vi "Read File.vi"(8 "error in (no error)":errorcluster, 11 "DAT in":refnum<class "Data.DAT.lvclass">) -> (0 "error out":errorcluster, 3 "DAT out":refnum<class "Data.DAT.lvclass">)   [LabVIEW 2016, in "Data.DAT.lvclass"]
uses:
  Data.DAT.lvclass
  C:/user/patrick/git/LV-to-ITX/src/Data/Data.lvclass
  Data/Data.lvclass/Data.ctl
  <vilib>/Utility/file.llb/Read Delimited Spreadsheet (string).vi
  Data/Data.lvclass
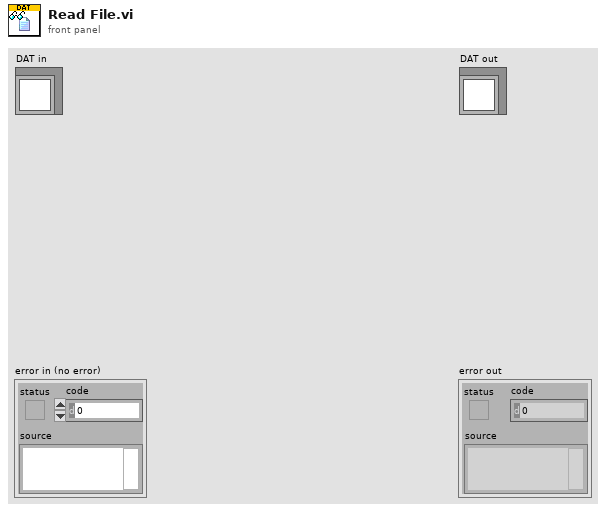
[diagram p1: front panel]
types:
  T1 = typedef "Data.lvclass/Dictionary--cluster.ctl" = cluster{"key":string, "value":variant}
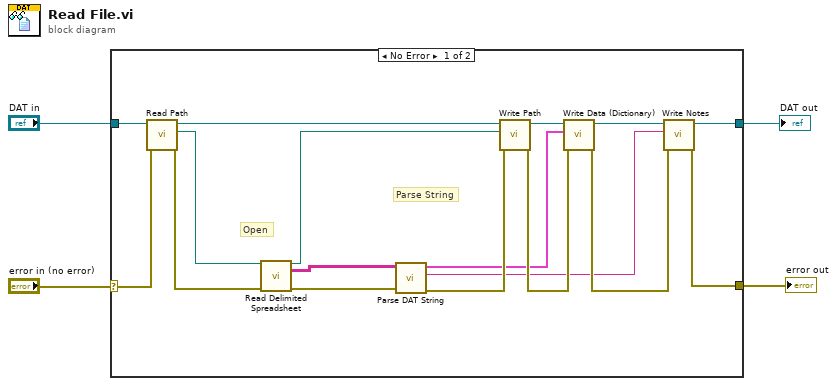
[diagram p0: block diagram]
diagram:
  n1 = case shown="No Error" "error in (no error)" {
    selector: "error in (no error)" -> [w5 w23]
    tunnel: "DAT in" -> [w8 w22]
    tunnel: [w7 w22] -> w3
    tunnel: [w6 w23] -> w2
    frame No Error {
      # "Parse String"
      # "Open"
      n2 = call "Read Path.vi"("error in (no error)"=w5, "Data Save"=w8) -> ("error out"=w20:errorcluster, "Path"=w10:path, "Data Save out"=w19:refnum<class "Data.DAT.lvclass">)  [unwired: 7 in]
      n3 = call-poly <vilib>:"Read Delimited Spreadsheet.vi"("file path (dialog if empty)"=w10, "error in (no error)"=w20) -> ("new file path (Not A Path if cancelled)"=w11:path, "all rows"=w9:string[][], "error out"=w21:errorcluster)  [unwired: 8 in, 3 out]
      n4 = call "Parse DAT String.vi"("error in (no error)"=w21, "spreadsheet string"=w9) -> ("error out"=w14:errorcluster, "Notes"=w12:string, "Data (Dictionary)"=w13:T1[])  [unwired: 7 in]
      n5 = call "Write Path.vi"("error in (no error)"=w14, "Path"=w11, "Data Save"=w19) -> ("error out"=w16:errorcluster, "Data Save out"=w18:refnum<class "Data.DAT.lvclass">)  [unwired: 7 in]
      n6 = call "Write Data (Dictionary).vi"("error in (no error)"=w16, "Data (Dictionary)"=w13, "Data Save"=w18) -> ("error out"=w15:errorcluster, "Data Save out"=w17:refnum<class "Data.DAT.lvclass">)  [unwired: 7 in]
      n7 = call "Write Notes.vi"("error in (no error)"=w15, "Notes"=w12, "Data Save"=w17) -> ("error out"=w6:errorcluster, "Data Save out"=w7:refnum<class "Data.DAT.lvclass">)  [unwired: 7 in]
    }
    frame Error {
    }
  }
  "error out" <- w2
  "DAT out" <- w3
